vi "Assert Same Type.vi"(7 "Message (\"\")":string, 8 "error in (no error)":errorcluster, 10 "Second":variant, 11 "First":variant) -> (0 "error out":errorcluster)   [LabVIEW 2017, in "Transparent Assertions.lvlib" / "Assertions.lvlib"]
doc: "Asserts that two values are of the same type. Returns an error if the assertion fails, and optionally appends a custom message to the error."
uses:
  Assertions.lvlib
  Constraints/Is Same Type/Is Same Type.lvclass
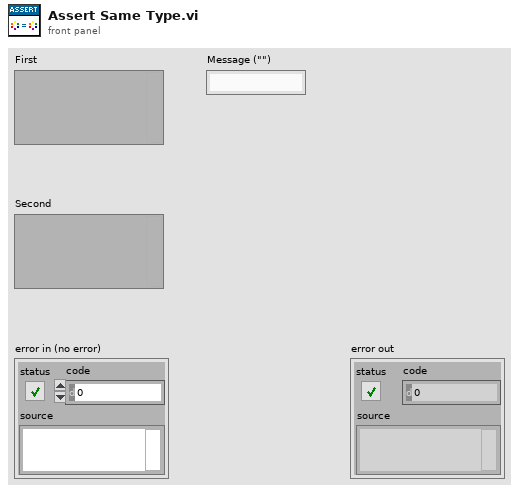
[diagram p1: front panel]
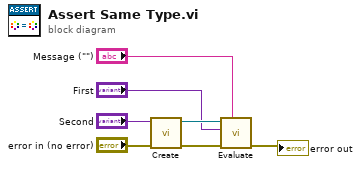
[diagram p0: block diagram]
diagram:
  n1 = call "Create.vi"("error in (no error)"="error in (no error)", "Expected"="Second") -> ("error out"=w6:errorcluster, "Is Same Type"=w3:refnum<class "Is Same Type.lvclass">)  [unwired: 8 in]
  n2 = call-dynamic "Evaluate.vi"("Message (\"\")"="Message (\"\")", "error in (no error)"=w6, "Actual"="First", "Constraint in"=w3) -> ("error out"=→"error out":errorcluster)  [unwired: 6 in, 1 out]
